vi "Get Virtual Instruments Attribute as JSON.vi"(8 "error in":errorcluster, 11 "Source":string) -> (0 "error out":errorcluster, 3 "<JSON>":string)   [LabVIEW 2024, in "Instrument Manager.lvclass"]
uses:
  Instrument Manager.lvclass
  Config from JSON/Config from JSON.lvclass
  D:/git/HAL/Source/Interfaces/IConfiguration/IConfiguration.lvclass
  Config from XML/Config from XML.lvclass
  Config from EXCEL/Config from EXCEL.lvclass
  Interfaces/IConfiguration/IConfiguration.lvclass
  <vilib>/JDP Science/JSONtext/JSONtext.lvlib
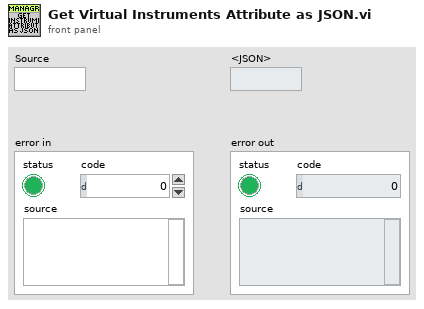
[diagram p1: front panel]
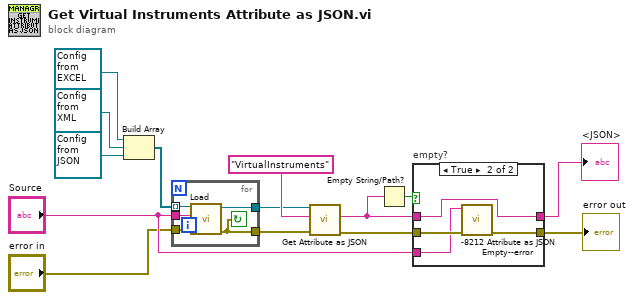
[diagram p0: block diagram]
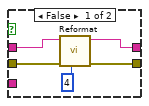
[diagram p2: hidden frame]
diagram:
  n1 = Build Array(refnum<class "Config from EXCEL.lvclass"> refnum ("Config from EXCEL.lvclass"), refnum<class "Config from XML.lvclass"> refnum ("Config from XML.lvclass"), refnum<class "Config from JSON.lvclass"> refnum ("Config from JSON.lvclass")) -> (w12:refnum<class "IConfiguration.lvclass">[])
  n2 = for {
    tunnel: w12 -> [w17] mode=indexing
    tunnel: "Source" -> [w19]
    tunnel: [w18] -> w13
    tunnel: [w16] -> w1
    tunnel: "error in" -> [w15]
    stop <- w16 continue-if-true
    n3 = call-dynamic "Load.vi"("error in"=w15, "Source"=w19, "IConfiguration in"=w17) -> ("error out"=w16:errorcluster, "IConfiguration out"=w18:refnum<class "IConfiguration.lvclass">)  [unwired: 7 in]
  }
  n4 = call-dynamic "Get Attribute as JSON.vi"("error in"=w1, "Attribute"="VirtualInstruments", "IConfiguration in"=w13) -> ("error out"=w7:errorcluster, "<JSON>"=w8:string)  [unwired: 6 in, 1 out]
  n5 = Empty String/Path?(string/path=w8) -> (empty?=w9:bool)
  n6 = case "empty?" shown="True" w9 {
    tunnel: w8 -> [w22 w28]
    tunnel: w7 -> [w24 w27]
    tunnel: [w23 w26] -> w6
    tunnel: [w21 w28] -> w5
    tunnel: "Source" -> [_ w25]
    frame False {
      n7 = call <vilib>:"Reformat.vi"("Pretty Print Levels"=4, "error in (no error)"=w24, "JSON"=w22) -> ("error out"=w23:errorcluster, "<JSON>"=w21:string)  [unwired: 5 in, 2 out]
    }
    frame True {
      n8 = call "-8212 Attribute as JSON Empty--error.vi"("error in"=w27, "Source"=w25) -> ("error out"=w26:errorcluster)  [unwired: 9 in]
    }
  }
  "<JSON>" <- w5
  "error out" <- w6
